vi "inches to encoder ticks.vi"(9 "Number of ticks in a rotation":dbl, 10 "Desired distance in inches":dbl, 11 "Wheel Diameter":dbl) -> (2 "Number of ticks needed to travel":dbl)   [LabVIEW 2014]
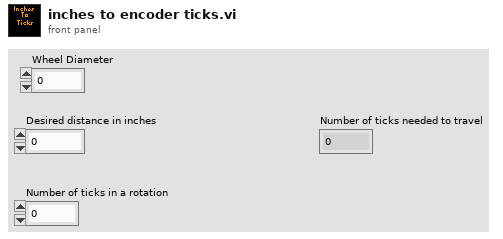
[diagram p1: front panel]
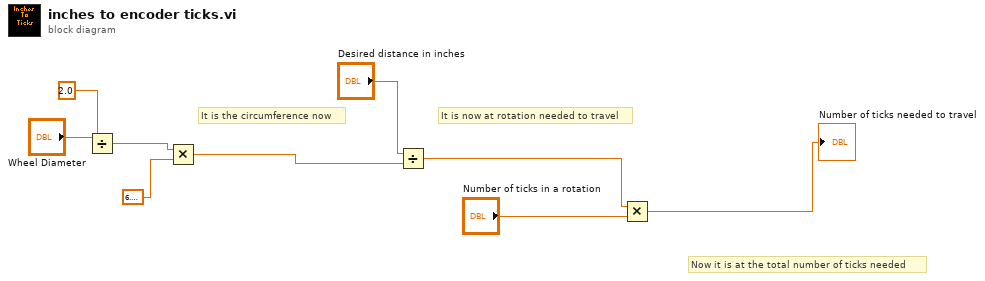
[diagram p0: block diagram]
diagram:
  # "Now it is at the total number of ticks needed"
  # "It is now at rotation needed to travel"
  # "It is the circumference now"
  n1 = Divide(x="Wheel Diameter", y=2.0) -> (x/y=w7:dbl)
  n2 = Multiply(x=w7, y=6.283185307179586) -> (x*y=w4:dbl)
  n3 = Divide(x="Desired distance in inches", y=w4) -> (x/y=w3:dbl)
  n4 = Multiply(x=w3, y="Number of ticks in a rotation") -> (x*y=→"Number of ticks needed to travel":dbl)
